vi "Helper - Elapsed Time.vi"() -> (0 "Frequency (Hz)":dbl, 3 "Time Elapsed (s)\nSince Last Iteration":dbl)   [LabVIEW 2011]
doc: "Calculates the amount of time that has passed since this subVI instance was last run (returns zero for the first run). Good for timing processes. Reentrant so that multiple copies can be used to time different things.\n\nBy Jason Curtis"
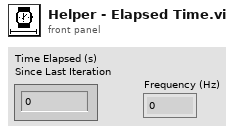
[diagram p1: front panel]
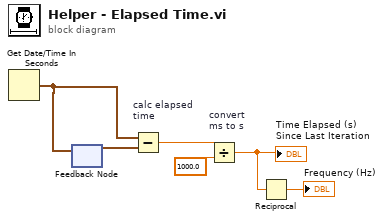
[diagram p0: block diagram]
diagram:
  n1 = Get Date/Time In Seconds() -> (seconds since 1Jan1904=w2:timestamp)
  n2 = feedback #1() -> (w3:timestamp)  [unwired: 1 in]
  n3 = feedback-in #1(w2) -> ()
  n4 = Subtract "calc elapsed\ntime"(x=w2, y=w3) -> (x-y=w1:dbl)
  n5 = Divide "convert\nms to s"(x=w1, y=1000.0) -> (x/y=w5:dbl)
  "Time Elapsed (s)\nSince Last Iteration" <- w5
  n6 = Reciprocal(x=w5) -> (1/x=→"Frequency (Hz)":dbl)
